vi "Get Subsystem from Alarm.vi"(8 "error in (no error)":errorcluster, 11 "Alarm URL":string) -> (0 "error out":errorcluster, 3 "Subsystem URL":refnum<k21>)   [LabVIEW 2024]
doc: "Gets the URL of the subsystem that includes the specified alarm."
uses:
  <resource>/objmgr/ni.var.rc
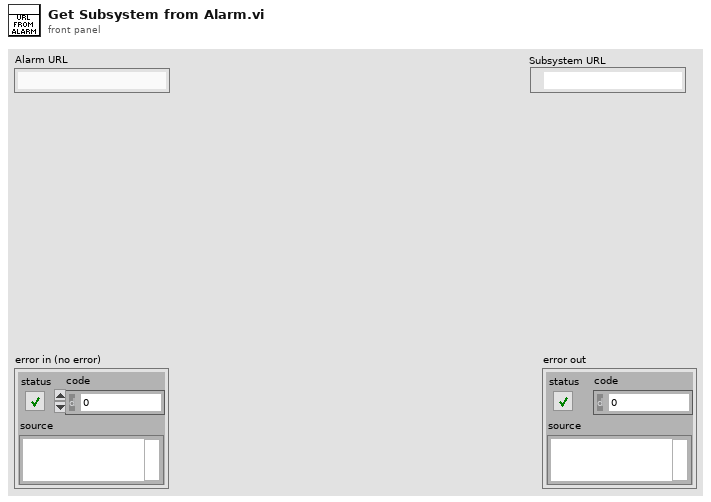
[diagram p1: front panel]
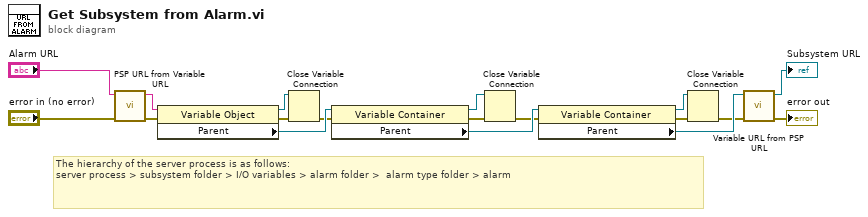
[diagram p0: block diagram]
diagram:
  # "The hierarchy of the server process is as follows:\nserver process > subsystem folder > I/O variables > alarm folder >  alarm type folder > alarm"
  n1 = call "PSP URL from Variable URL.vi"("error in (no error)"="error in (no error)", "Shared Variable URL"="Alarm URL") -> ("error out"=w14:errorcluster, "PSP URL"=w10:string)  [unwired: 8 in]
  n2 = property class="Variable Object"(reference=w10, error in=w14) -> (reference out=w5:refnum<k21>, error out=w16:errorcluster, "Parent"=w11:refnum<k21>)
  n3 = Close Variable Connection(8:w16, 11:w5) -> (0:w6:errorcluster)
  n4 = property class="Variable Container"(reference=w11, error in=w6) -> (reference out=w3:refnum<k21>, error out=w18:errorcluster, "Parent"=w17:refnum<k21>)
  n5 = Close Variable Connection(8:w18, 11:w3) -> (0:w4:errorcluster)
  n6 = property class="Variable Container"(reference=w17, error in=w4) -> (reference out=w1:refnum<k21>, error out=w13:errorcluster, "Parent"=w9:refnum<k21>)
  n7 = Close Variable Connection(8:w13, 11:w1) -> (0:w2:errorcluster)
  n8 = call "Variable URL from PSP URL.vi"("error in (no error)"=w2, "PSP URL"=w9) -> ("error out"=→"error out":errorcluster, "Shared Variable URL"=→"Subsystem URL":refnum<k21>)  [unwired: 8 in]
